vi "IEPE - Continuous Input - FFT -save.vi"() -> ()   [LabVIEW 2022 SP3]
doc: "This example demonstrates how to continuously acquire buffered acceleration, sound pressure, or force measurements from IEPE sensors using a DAQmx device.\n\nFor instructions on how to connect your signals to the DAQ device, refer to your device documentation."
uses:
  <vilib>/Utility/error.llb/DialogType.ctl
  <vilib>/DAQmx/read.llb/DAQmx Read (Analog Wfm 1Chan NSamp).vi
  <vilib>/DAQmx/create/channels.llb/DAQmx Create Channel (AI-Acceleration-Accelerometer).vi
  <vilib>/DAQmx/configure/timing.llb/DAQmx Timing (Sample Clock).vi
  <vilib>/DAQmx/configure/task.llb/DAQmx Configure Logging (TDMS).vi
  <vilib>/DAQmx/configure/trigger.llb/DAQmx Start Trigger (Digital Edge).vi
  <vilib>/DAQmx/configure/trigger.llb/DAQmx Start Trigger (Time).vi
  <vilib>/DAQmx/configure/trigger.llb/DAQmx Start Trigger (Analog Edge).vi
  <vilib>/DAQmx/miscellaneous.llb/DAQmx Fill In Error Info.vi
  <vilib>/measure/maspectr.llb/FFT Spectrum (Mag-Phase) for 1 Chan.vi
  <resource>/objmgr/daqmx.rc
  <vilib>/measure/NI_MAPro.lvlib
panel:
  in  "Enum":T1(ring)
  out "Phase":cluster{"f0":dbl, "df":dbl, "magnitude":dbl[]}(graph)
  out "Mag":cluster{"f0":dbl, "df":dbl, "phase":dbl[]}(graph)
  in  "Window":dbl
  in  "Restart Aaveraging":bool
  in  "Trigger Type":T2(tab)
  in  "Digital Start Trigger Edge":i32(ring)=10280 caption="Edge" items=["Rising"=10280, "Falling"=10171]
  in  "Digital Start Trigger Source":tag="/Dev1/PFI0" caption="Source"
  in  "Digital Pause Trigger Pause When":i32(ring)=10192 caption="Pause When" items=["High"=10192, "Low"=10214]
  in  "Digital Pause Trigger Source":tag="/Dev1/PFI0" caption="Source"
  in  "Analog Start Trigger Level":dbl caption="Level" format="%0.2f"
  in  "Analog Start Trigger Hysteresis":dbl caption="Hysteresis" format="%.2f"
  in  "Analog Start Trigger Slope":i32(ring)=10280 caption="Slope" items=["Rising"=10280, "Falling"=10171]
  in  "Analog Start Trigger Source":string="APFI0" caption="Source"
  in  "Analog Pause Trigger Source":string="APFI0" caption="Source"
  in  "Analog Pause Trigger Pause When":i32(ring)=10093 caption="Pause When" items=["Above Level"=10093, "Below Level"=10107]
  in  "Analog Pause Trigger Level":dbl caption="Level" format="%.2f"
  in  "When":timestamp
  in  "Select Time\nManually":bool
  in  "Stop":bool
  out "Waveform Graph":waveform(dbl)(graph)
  in  "TDMS File Path":path
  in  "Samples per Loop":i32=1000
  in  "Sample Rate":dbl=1000.0
  in  "Sample Clock Source":tag="OnboardClock"
  out "Actual Sample Rate":dbl=1000.0000111176631 format="%0.2f"
  in  "Logging Mode":i32(ring)=10231 items=["Off"=10231, "Log and Read"=15842]
  # "Time Domain"
  # "Timing Settings"
  # "FFT Magnitude"
  # "FFT\nParamters"
  # "Logging Settings"
  # "FFT Phase"
  # "Trigger Settings"
  # "To enable triggers, select a tab above, and configure the settings.\n\nNot all hardware supports all trigger types. Refer to your device documentation for more information."
  # "This trigger type is not supported in continuous sample timing. \n\nRefer to your device documentation for more information on which triggers are supported."
  # "This trigger type is not supported in continuous sample timing. \n\nRefer to your device documentation for more information on which triggers are supported."
  # "If time is not manually set, task will begin after 10 seconds"
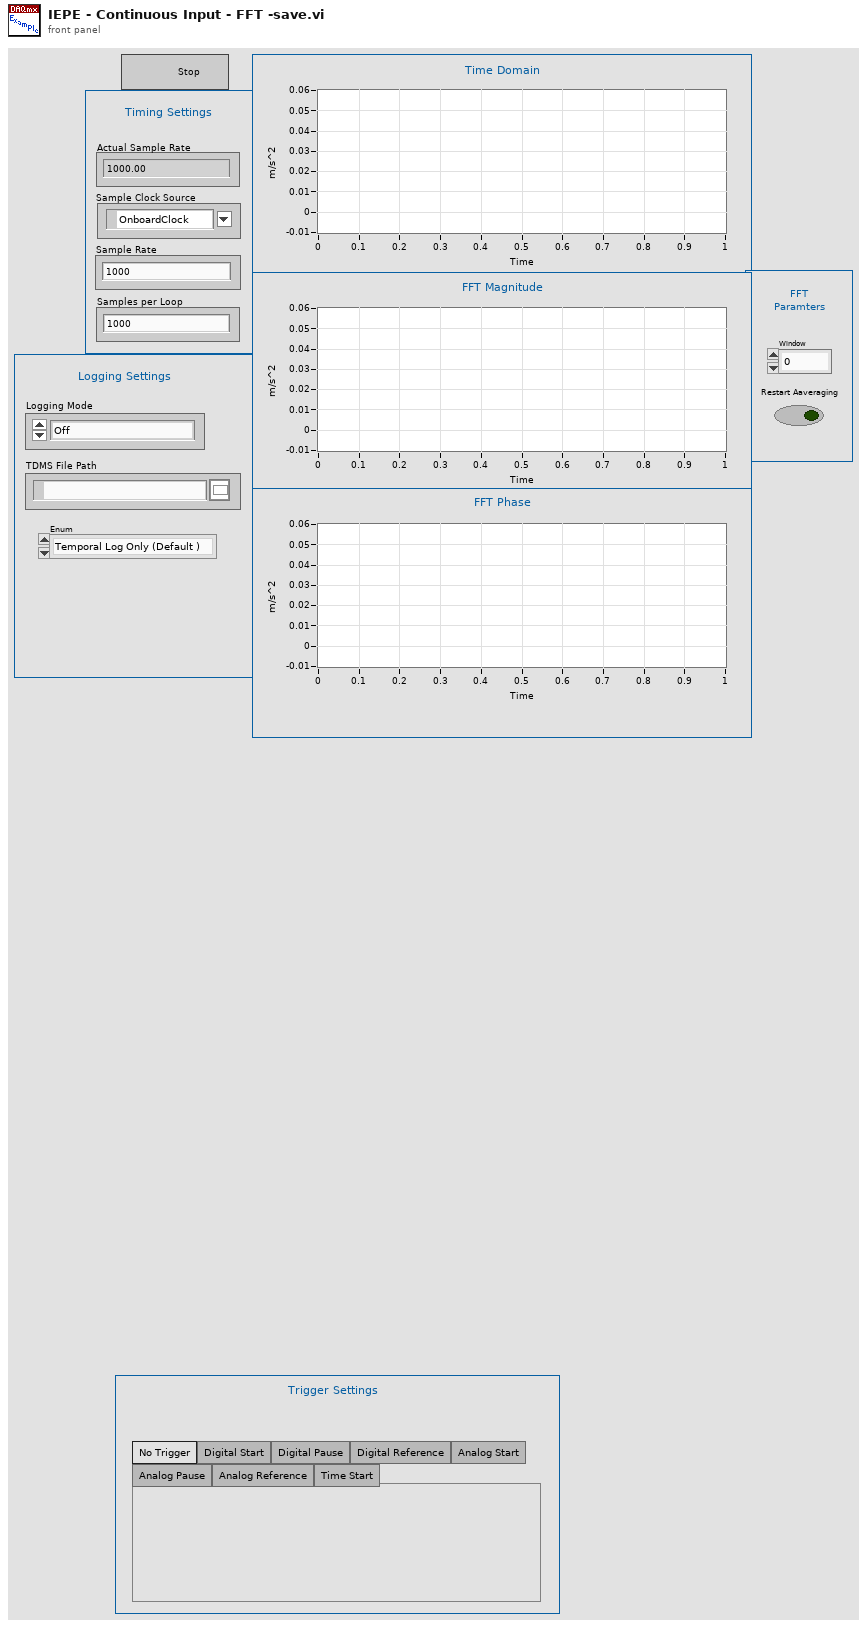
[diagram p1: front panel]
types:
  T1 = enum16{"Temporal Log Only (Default )", "FFT Log Only", "Temporal and FFT Log"}
  T2 = enum32{"No Trigger", "Digital Start", "Digital Pause", "Digital Reference", "Analog Start", "Analog Pause", "Analog Reference", "Time Start"}
  T3 = typedef "DialogType.ctl" = u16
  T4 = enum16{"open", "replace", "create", "open or create", "replace or create", "replace or create with confirmation"}
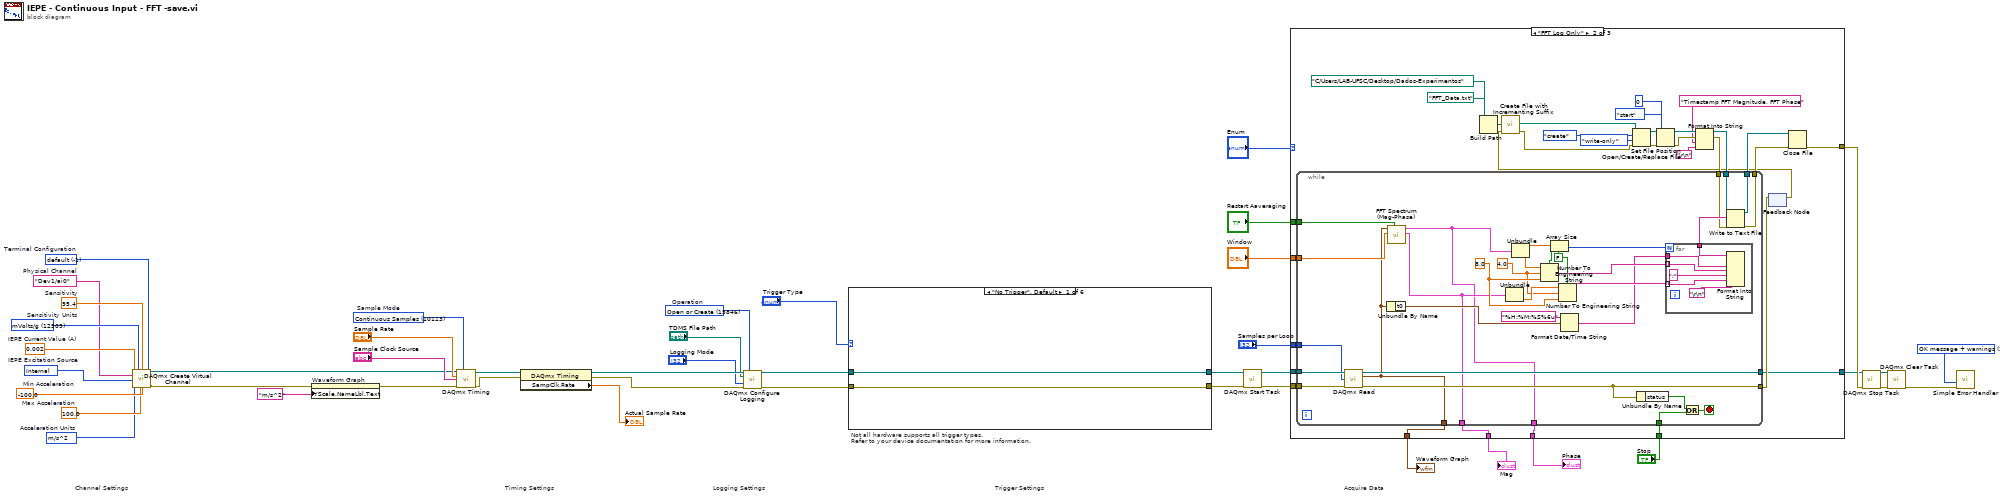
[diagram p0: block diagram]
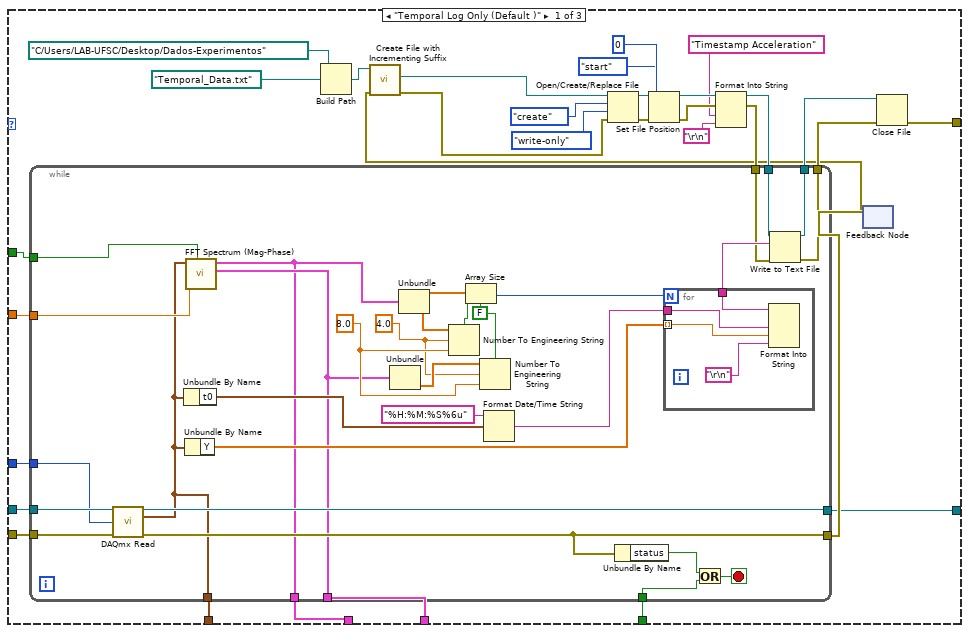
[diagram p2: hidden frame]
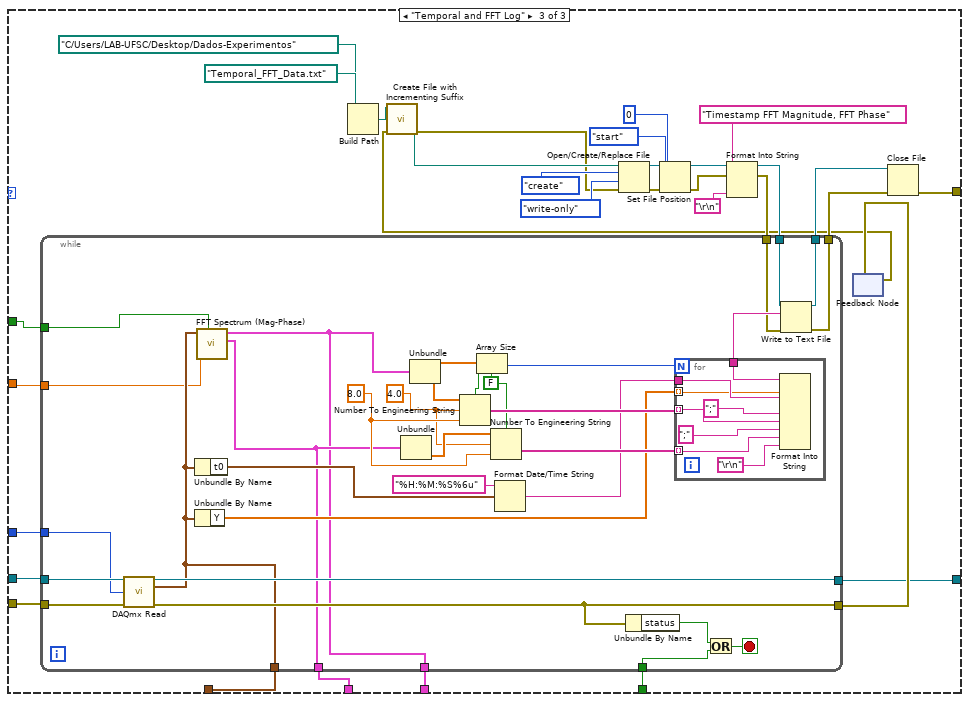
[diagram p3: hidden frame]
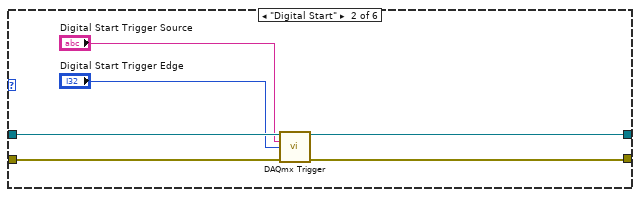
[diagram p4: hidden frame]
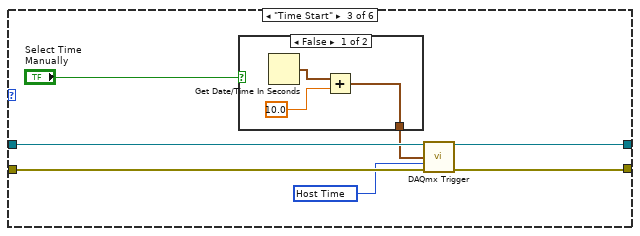
[diagram p5: hidden frame]
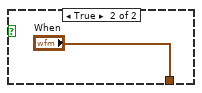
[diagram p6: hidden frame]
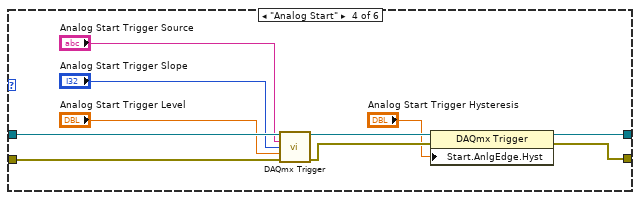
[diagram p7: hidden frame]
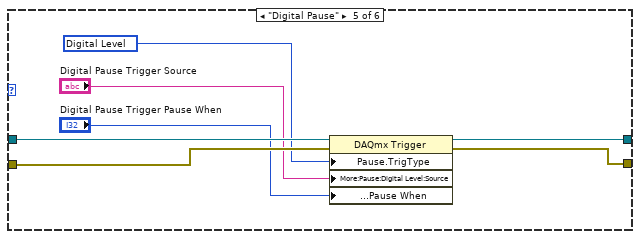
[diagram p8: hidden frame]
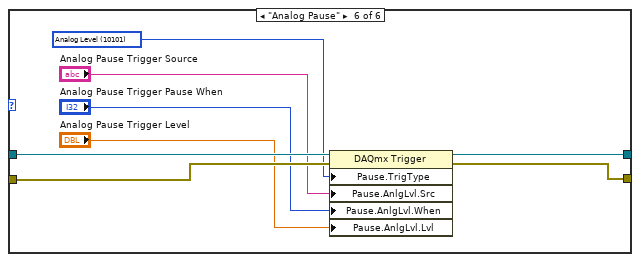
[diagram p9: hidden frame]
diagram:
  w22 = 100.0  # Max Acceleration
  w23 = -100.0  # Min Acceleration
  w16 = -1 items=["default"=-1, "RSE"=10083, "NRSE"=10078, "Differential"=10106, "Pseudodifferential"=12529]  # Terminal Configuration
  w13 = tag "Dev1/ai0"  # Physical Channel
  w18 = 0.002  # IEPE Current Value (A)
  w19 = 10200 items=["Internal"=10200, "External"=10167, "None"=10230]  # IEPE Excitation Source
  w17 = 12470 items=["g"=10186, "m/s^2"=12470, "in/s^2"=12471, "From Custom Scale"=10065]  # Acceleration Units
  w20 = 12509 items=["mVolts/g"=12509, "Volts/g"=12510]  # Sensitivity Units
  w21 = 95.4  # Sensitivity
  w24 = T3 3 items=["no dialog", "OK message", "continue or stop message", "OK message + warnings", "continue/stop + warnings"] ("type of dialog (OK msg:1)")
  w40 = 15846 items=["Open"=10437, "Open or Create"=15846, "Create or Replace"=15847, "Create"=15848]  # Operation
  w43 = 10123 items=["Finite Samples"=10178, "Continuous Samples"=10123, "Hardware Timed Single Point"=12522]  # Sample Mode
  # "Trigger Settings"
  # "Not all hardware supports all trigger types.\nRefer to your device documentation for more information."
  # "Acquire Data"
  # "Timing Settings"
  # "Channel Settings"
  # "Logging Settings"
  n1 = call-poly <vilib>:"DAQmx Create Virtual Channel.vi"("maximum value"=w22, "minimum value"=w23, "input terminal configuration"=w16, "physical channels"=w13, "current excitation source"=w19, "current excitation value"=w18, "units"=w17, "sensitivity"=w21, "sensitivity units"=w20) -> ("task out"=w14:refnum<k21>, "error out"=w15:errorcluster)  [unwired: 5 in]
  n2 = property on="Waveform Graph" class="WFGraph (strict)"(error in=w15, "YScale.NameLbl.Text"="m/s^2") -> (error out=w34:errorcluster)  [unwired: 1 in, 1 out]
  n3 = call-poly <vilib>:"DAQmx Timing.vi"("task/channels in"=w14, "sample mode"=w43, "rate"="Sample Rate", "source"="Sample Clock Source", "error in"=w34) -> ("task out"=w45:refnum<k21>, "error out"=w44:errorcluster)  [unwired: 9 in]
  n4 = property class="DAQmx Timing"(reference=w45, error in=w44) -> (reference out=w42:refnum<k21>, error out=w41:errorcluster, "SampClk.Rate"=→"Actual Sample Rate":dbl)
  n5 = call-poly <vilib>:"DAQmx Configure Logging.vi"("task/channels in"=w42, "operation"=w40, "file path"="TDMS File Path", "logging mode"="Logging Mode", "error in"=w41) -> ("task out"=w29:refnum<k21>, "error out"=w30:errorcluster)  [unwired: 9 in]
  n6 = case shown="\"No Trigger\", Default" "Trigger Type" {
    tunnel: w29 -> [w47 w53 w60 w74 w81 w89]
    tunnel: w30 -> [w46 w52 w59 w73 w78 w86]
    tunnel: [w47 w51 w58 w71 w80 w88] -> w27
    tunnel: [w46 w50 w57 w70 w79 w87] -> w28
    frame "No Trigger", Default {
    }
    frame "Digital Start" {
      n7 = call-poly <vilib>:"DAQmx Trigger.vi"("task/channels in"=w53, "source"="Digital Start Trigger Source", "edge"="Digital Start Trigger Edge", "error in"=w52) -> ("task out"=w51:refnum<k21>, "error out"=w50:errorcluster)  [unwired: 10 in]
    }
    frame "Time Start" {
      w54 = 16126 items=["Host Time"=16126, "I/O Device Time"=16127] ("timescale")
      n8 = case shown="False" "Select Time\nManually" {
        tunnel: [w62 "When"] -> w55
        frame False {
          n9 = Get Date/Time In Seconds() -> (seconds since 1Jan1904=w63:timestamp)
          n10 = Add(x=w63, y=10.0) -> (x+y=w62:timestamp)
        }
        frame True {
        }
      }
      n11 = call-poly <vilib>:"DAQmx Trigger.vi"("task/channels in"=w60, "when"=w55, "timescale"=w54, "error in"=w59) -> ("task out"=w58:refnum<k21>, "error out"=w57:errorcluster)  [unwired: 10 in]
    }
    frame "Analog Start" {
      n12 = call-poly <vilib>:"DAQmx Trigger.vi"("task/channels in"=w74, "source"="Analog Start Trigger Source", "slope"="Analog Start Trigger Slope", "level"="Analog Start Trigger Level", "error in"=w73) -> ("task out"=w69:refnum<k21>, "error out"=w68:errorcluster)  [unwired: 9 in]
      n13 = property class="DAQmx Trigger"(reference=w69, error in=w68, "Start.AnlgEdge.Hyst"="Analog Start Trigger Hysteresis") -> (reference out=w71:refnum<k21>, error out=w70:errorcluster)
    }
    frame "Digital Pause" {
      w77 = 10152 items=["Analog Level"=10101, "Analog Window"=10103, "Digital Level"=10152, "Digital Pattern"=10398, "None"=10230] ("Pause.TrigType")
      n14 = property class="DAQmx Trigger"(reference=w81, error in=w78, "Pause.TrigType"=w77, "More:Pause:Digital Level:Source"="Digital Pause Trigger Source", "More:Pause:Digital Level:Pause When"="Digital Pause Trigger Pause When") -> (reference out=w80:refnum<k21>, error out=w79:errorcluster)
    }
    frame "Analog Pause" {
      w85 = 10101 items=["Analog Level"=10101, "Analog Window"=10103, "Digital Level"=10152, "Digital Pattern"=10398, "None"=10230] ("Pause.TrigType")
      n15 = property class="DAQmx Trigger"(reference=w89, error in=w86, "Pause.TrigType"=w85, "Pause.AnlgLvl.Src"="Analog Pause Trigger Source", "Pause.AnlgLvl.When"="Analog Pause Trigger Pause When", "Pause.AnlgLvl.Lvl"="Analog Pause Trigger Level") -> (reference out=w88:refnum<k21>, error out=w87:errorcluster)
    }
  }
  n16 = call <vilib>:"DAQmx Start Task.vi"("task/channels in"=w27, "error in"=w28) -> ("task out"=w26:refnum<k21>, "error out"=w25:errorcluster)  [unwired: 12 in]
  n17 = case shown="\"FFT Log Only\"" "Enum" {
    tunnel: w26 -> [w107 w185 w236]
    tunnel: w25 -> [w106 w184 w235]
    tunnel: [w105 w168 w234] -> w10
    tunnel: [w103 w167 w233] -> w8
    tunnel: "Samples per Loop" -> [w102 w166 w232]
    tunnel: "Window" -> [w100 w165 w224]
    tunnel: "Restart Aaveraging" -> [w99 w164 w223]
    tunnel: "Stop" -> [w101 w163 w231]
    tunnel: [w98 w162 w230] -> w3
    tunnel: [w91 w154 w221] -> w2
    tunnel: [w90 w155 w222] -> w1
    frame "Temporal Log Only (Default )" {
      n18 = Build Path(base path=path "C:/Users/LAB-UFSC/Desktop/Dados-Experimentos", name or relative path=path "Temporal_Data.txt" ("default name")) -> (appended path=w96:path)
      n19 = feedback #1() -> (w93:errorcluster)  [unwired: 1 in]
      n20 = call <vilib>:"Create File with Incrementing Suffix.vi"("error in (no error)"=w93, "file path"=w96) -> ("error out"=w92:errorcluster, "actual path"=w94:path)  [unwired: 7 in, 1 out]
      n21 = Open/Create/Replace File(file path (use dialog)=w94, error in=w92, operation (0:open)=T4."create", access (0:read/write)=enum16{"read/write", "read-only", "write-only"}."write-only") -> (refnum out=w119:refnum<file>, error out=w120:errorcluster)  [unwired: 2 in, 1 out]
      n22 = Set File Position(offset (in bytes) (0)=i64 0, refnum=w119, from (0:start)=enum16{"start", "end", "current"}."start", error in=w120) -> (refnum out=w112:refnum<file>, error out=w113:errorcluster)
      n23 = Format Into String(initial string=w112, error in=w113, "Timestamp Acceleration", "\r\n") -> (resulting string=w110:refnum<file>, error out=w111:errorcluster)  [unwired: 1 in]
      n24 = while {
        tunnel: w107 -> [w135]
        tunnel: w106 -> [w136]
        tunnel: [w148] -> w103
        tunnel: [w134] -> w104
        tunnel: [w139] -> w115
        tunnel: w111 -> [w138]
        tunnel: [w137] -> w114
        tunnel: w110 -> [w130]
        tunnel: w102 -> [w128]
        tunnel: w101 -> [w127]
        tunnel: w100 -> [w126]
        tunnel: w99 -> [w125]
        tunnel: [w124] -> w98
        tunnel: [w123] -> w91
        tunnel: [w122] -> w90
        stop <- w147 stop-if-true
        w142 = 8.0 ("Precision")
        w141 = 4.0 ("Width")
        w143 = FALSE ("use system decimal point (T)")
        n25 = call-poly <vilib>:"DAQmx Read.vi"("task/channels in"=w135, "number of samples per channel"=w128, "error in"=w136) -> ("task out"=w148:refnum<k21>, "data"=w124:waveform(dbl), "error out"=w134:errorcluster)  [unwired: 10 in]
        n26 = Unbundle By Name(w124) -> ("t0"=w133:timestamp)
        n27 = Unbundle By Name(w124) -> ("Y"=w129:dbl[])
        n28 = call-poly <vilib>:"FFT Spectrum (Mag-Phase).vi"("restart averaging (F)"=w125, "window"=w126, "time signal"=w124) -> ("phase"=w123:cluster{"f0":dbl, "df":dbl, "phase":dbl[]}, "magnitude"=w122:cluster{"f0":dbl, "df":dbl, "magnitude":dbl[]})  [unwired: 4 in, 3 out]
        n29 = Unbundle(w123) -> ("phase"=w146:dbl[])  [unwired: 2 out]
        n30 = Unbundle(w122) -> ("magnitude"=w144:dbl[])  [unwired: 2 out]
        n31 = Number To Engineering String(1:w143, 2:w142, 3:w141, 4:w144) -> ()  [unwired: 1 out]
        n32 = Array Size(array=w144) -> (size(s)=w145:i32)
        n33 = Number To Engineering String(1:w143, 2:w142, 3:w141, 4:w146) -> ()  [unwired: 1 out]
        n34 = Format Date/Time String(time format string (%c)="%H:%M:%S%6u", seconds (now)=w133) -> (date/time string=w132:string)  [unwired: 1 in]
        n35 = Unbundle By Name(w134) -> ("status"=w149:bool)
        n36 = for {
          N: w145 -> [_]
          tunnel: [w153] -> w140
          tunnel: w129 -> [w152] mode=indexing
          tunnel: w132 -> [w151]
          n37 = Format Into String(w151, w152, "\r\n") -> (resulting string=w153:string)  [unwired: 3 in, 1 out]
        }
        n38 = Or(x=w149, y=w127) -> (x .or. y?=w147:bool)
        n39 = Write to Text File(file (use dialog)=w130, text=w140, error in=w138) -> (refnum out=w139:refnum<file>, error out=w137:errorcluster)  [unwired: 1 in, 1 out]
      }
      n40 = feedback-in #1(w104) -> ()
      n41 = Close File(refnum=w115, error in=w114) -> (error out=w105:errorcluster)  [unwired: 1 out]
    }
    frame "FFT Log Only" {
      n42 = Build Path(base path=path "C:/Users/LAB-UFSC/Desktop/Dados-Experimentos", name or relative path=path "FFT_Data.txt" ("default name")) -> (appended path=w160:path)
      n43 = feedback #2() -> (w157:errorcluster)  [unwired: 1 in]
      n44 = call <vilib>:"Create File with Incrementing Suffix.vi"("error in (no error)"=w157, "file path"=w160) -> ("error out"=w156:errorcluster, "actual path"=w158:path)  [unwired: 7 in, 1 out]
      n45 = Open/Create/Replace File(file path (use dialog)=w158, error in=w156, operation (0:open)=T4."create", access (0:read/write)=enum16{"read/write", "read-only", "write-only"}."write-only") -> (refnum out=w181:refnum<file>, error out=w182:errorcluster)  [unwired: 2 in, 1 out]
      n46 = Set File Position(offset (in bytes) (0)=i64 0, refnum=w181, from (0:start)=enum16{"start", "end", "current"}."start", error in=w182) -> (refnum out=w174:refnum<file>, error out=w175:errorcluster)
      n47 = Format Into String(initial string=w174, error in=w175, "Timestamp FFT Magnitude, FFT Phase", "\r\n") -> (resulting string=w172:refnum<file>, error out=w173:errorcluster)  [unwired: 1 in]
      n48 = while {
        tunnel: w185 -> [w199]
        tunnel: w184 -> [w200]
        tunnel: [w198] -> w169
        tunnel: [w203] -> w177
        tunnel: w173 -> [w202]
        tunnel: [w201] -> w176
        tunnel: w172 -> [w194]
        tunnel: [w193] -> w167
        tunnel: w166 -> [w192]
        tunnel: w165 -> [w191]
        tunnel: w164 -> [w190]
        tunnel: w163 -> [w189]
        tunnel: [w188] -> w162
        tunnel: [w187] -> w155
        tunnel: [w186] -> w154
        stop <- w213 stop-if-true
        w206 = 8.0 ("Precision")
        w205 = 4.0 ("Width")
        w207 = FALSE ("use system decimal point (T)")
        n49 = call-poly <vilib>:"DAQmx Read.vi"("task/channels in"=w199, "number of samples per channel"=w192, "error in"=w200) -> ("task out"=w193:refnum<k21>, "data"=w188:waveform(dbl), "error out"=w198:errorcluster)  [unwired: 10 in]
        n50 = Unbundle By Name(w188) -> ("t0"=w197:timestamp)
        n51 = call-poly <vilib>:"FFT Spectrum (Mag-Phase).vi"("restart averaging (F)"=w190, "window"=w191, "time signal"=w188) -> ("phase"=w187:cluster{"f0":dbl, "df":dbl, "phase":dbl[]}, "magnitude"=w186:cluster{"f0":dbl, "df":dbl, "magnitude":dbl[]})  [unwired: 4 in, 3 out]
        n52 = Unbundle(w187) -> ("phase"=w211:dbl[])  [unwired: 2 out]
        n53 = Unbundle(w186) -> ("magnitude"=w208:dbl[])  [unwired: 2 out]
        n54 = Number To Engineering String(1:w207, 2:w206, 3:w205, 4:w208) -> (0:w210:string[])
        n55 = Array Size(array=w208) -> (size(s)=w209:i32)
        n56 = Number To Engineering String(1:w207, 2:w206, 3:w205, 4:w211) -> (0:w212:string[])
        n57 = Format Date/Time String(time format string (%c)="%H:%M:%S%6u", seconds (now)=w197) -> (date/time string=w196:string)  [unwired: 1 in]
        n58 = Unbundle By Name(w198) -> ("status"=w214:bool)
        n59 = for {
          N: w209 -> [_]
          tunnel: [w220] -> w204
          tunnel: w210 -> [w216] mode=indexing
          tunnel: w212 -> [w218] mode=indexing
          tunnel: w196 -> [w215]
          n60 = Format Into String(w215, w216, ";", w218, "\r\n") -> (resulting string=w220:string)  [unwired: 3 in, 1 out]
        }
        n61 = Or(x=w214, y=w189) -> (x .or. y?=w213:bool)
        n62 = Write to Text File(file (use dialog)=w194, text=w204, error in=w202) -> (refnum out=w203:refnum<file>, error out=w201:errorcluster)  [unwired: 1 in, 1 out]
      }
      n63 = feedback-in #2(w169) -> ()
      n64 = Close File(refnum=w177, error in=w176) -> (error out=w168:errorcluster)  [unwired: 1 out]
    }
    frame "Temporal and FFT Log" {
      n65 = Build Path(base path=path "C:/Users/LAB-UFSC/Desktop/Dados-Experimentos", name or relative path=path "Temporal_FFT_Data.txt" ("default name")) -> (appended path=w229:path)
      n66 = feedback #3() -> (w226:errorcluster)  [unwired: 1 in]
      n67 = call <vilib>:"Create File with Incrementing Suffix.vi"("error in (no error)"=w226, "file path"=w229) -> ("error out"=w225:errorcluster, "actual path"=w227:path)  [unwired: 7 in, 1 out]
      n68 = Open/Create/Replace File(file path (use dialog)=w227, error in=w225, operation (0:open)=T4."create", access (0:read/write)=enum16{"read/write", "read-only", "write-only"}."write-only") -> (refnum out=w246:refnum<file>, error out=w245:errorcluster)  [unwired: 2 in, 1 out]
      n69 = Set File Position(offset (in bytes) (0)=i64 0, refnum=w246, from (0:start)=enum16{"start", "end", "current"}."start", error in=w245) -> (refnum out=w250:refnum<file>, error out=w249:errorcluster)
      n70 = Format Into String(initial string=w250, error in=w249, "Timestamp FFT Magnitude, FFT Phase", "\r\n") -> (resulting string=w252:refnum<file>, error out=w251:errorcluster)  [unwired: 1 in]
      n71 = while {
        tunnel: w236 -> [w266]
        tunnel: w235 -> [w267]
        tunnel: [w281] -> w233
        tunnel: [w265] -> w237
        tunnel: [w270] -> w247
        tunnel: w251 -> [w269]
        tunnel: [w268] -> w248
        tunnel: w252 -> [w261]
        tunnel: w232 -> [w259]
        tunnel: w231 -> [w258]
        tunnel: [w257] -> w230
        tunnel: w224 -> [w256]
        tunnel: w223 -> [w255]
        tunnel: [w254] -> w222
        tunnel: [w253] -> w221
        stop <- w280 stop-if-true
        w273 = 8.0 ("Precision")
        w272 = 4.0 ("Width")
        w274 = FALSE ("use system decimal point (T)")
        n72 = call-poly <vilib>:"DAQmx Read.vi"("task/channels in"=w266, "number of samples per channel"=w259, "error in"=w267) -> ("task out"=w281:refnum<k21>, "data"=w257:waveform(dbl), "error out"=w265:errorcluster)  [unwired: 10 in]
        n73 = Unbundle By Name(w257) -> ("t0"=w264:timestamp)
        n74 = Unbundle By Name(w257) -> ("Y"=w260:dbl[])
        n75 = call-poly <vilib>:"FFT Spectrum (Mag-Phase).vi"("restart averaging (F)"=w255, "window"=w256, "time signal"=w257) -> ("phase"=w254:cluster{"f0":dbl, "df":dbl, "phase":dbl[]}, "magnitude"=w253:cluster{"f0":dbl, "df":dbl, "magnitude":dbl[]})  [unwired: 4 in, 3 out]
        n76 = Unbundle(w254) -> ("phase"=w278:dbl[])  [unwired: 2 out]
        n77 = Unbundle(w253) -> ("magnitude"=w275:dbl[])  [unwired: 2 out]
        n78 = Number To Engineering String(1:w274, 2:w273, 3:w272, 4:w275) -> (0:w277:string[])
        n79 = Array Size(array=w275) -> (size(s)=w276:i32)
        n80 = Number To Engineering String(1:w274, 2:w273, 3:w272, 4:w278) -> (0:w279:string[])
        n81 = Format Date/Time String(time format string (%c)="%H:%M:%S%6u", seconds (now)=w264) -> (date/time string=w263:string)  [unwired: 1 in]
        n82 = Unbundle By Name(w265) -> ("status"=w282:bool)
        n83 = for {
          N: w276 -> [_]
          tunnel: [w290] -> w271
          tunnel: w277 -> [w285] mode=indexing
          tunnel: w279 -> [w287] mode=indexing
          tunnel: w263 -> [w289]
          tunnel: w260 -> [w283] mode=indexing
          n84 = Format Into String(w289, w283, ";", w285, ";", w287, "\r\n") -> (resulting string=w290:string)  [unwired: 3 in, 1 out]
        }
        n85 = Or(x=w282, y=w258) -> (x .or. y?=w280:bool)
        n86 = Write to Text File(file (use dialog)=w261, text=w271, error in=w269) -> (refnum out=w270:refnum<file>, error out=w268:errorcluster)  [unwired: 1 in, 1 out]
      }
      n87 = feedback-in #3(w237) -> ()
      n88 = Close File(refnum=w247, error in=w248) -> (error out=w234:errorcluster)  [unwired: 1 out]
    }
  }
  "Waveform Graph" <- w3
  "Phase" <- w2
  "Mag" <- w1
  n89 = call <vilib>:"DAQmx Stop Task.vi"("task/channels in"=w8, "error in"=w10) -> ("task out"=w33:refnum<k21>, "error out"=w32:errorcluster)  [unwired: 12 in]
  n90 = call <vilib>:"DAQmx Clear Task.vi"("task in"=w33, "error in"=w32) -> ("error out"=w11:errorcluster)  [unwired: 13 in]
  n91 = call <vilib>:"Simple Error Handler.vi"("type of dialog (OK msg:1)"=w24, "error in (no error)"=w11) -> ()  [unwired: 3 in, 5 out]
